vi "SigProc_subVI createPyCode.vi"(0 "newScriptCode":string) -> (1 "scriptStartIdx":i32, 2 "pyCode":string)   [LabVIEW 2018, in "Sig2MS.lvclass"]
uses:
  Sig2MS.lvclass
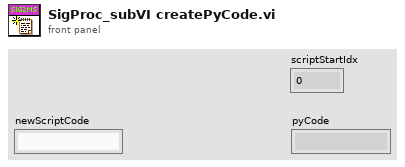
[diagram p1: front panel]
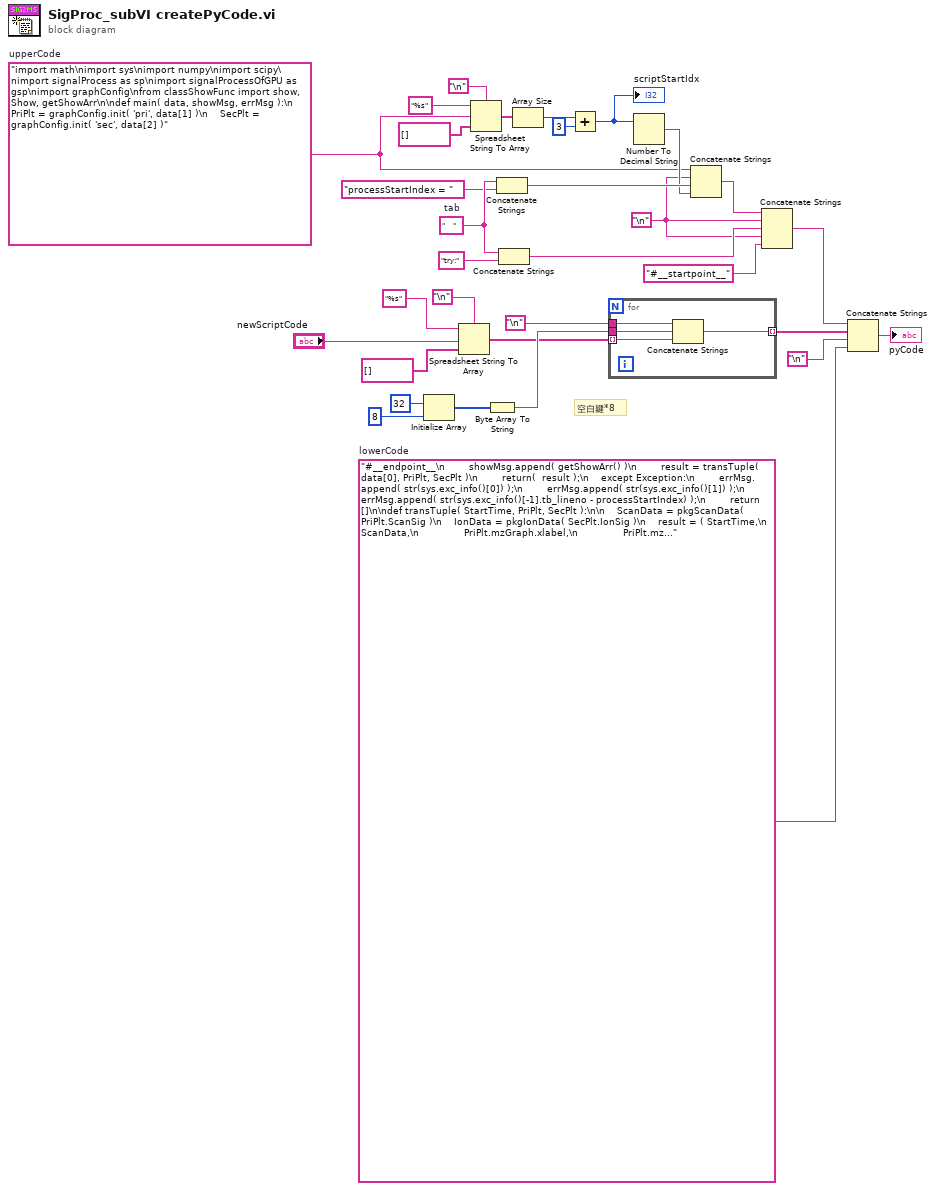
[diagram p0: block diagram]
diagram:
  w14 = "    "  # tab
  w6 = "\n"
  w5 = "#__endpoint__\n        showMsg.append( getShowArr() )\n        result = transTuple( data[0], PriPlt, SecPlt )\n        return(  result );\n    except Exception:\n        errMsg.append( str(sys.exc_info()[0]) );\n        errMsg.append( str(sys.exc_info()[1]) );\n        errMsg.append( str(sys.exc_info()[-1].tb_lineno - processStartIndex) );\n        return []\n\ndef transTuple( StartTime, PriPlt, SecPlt ):\n\n    ScanData = pkgScanData( PriPlt.ScanSig )\n    IonData = pkgIonData( SecPlt.IonSig )\n    result = ( StartTime,\n               ScanData,\n               PriPlt.mzGraph.xlabel,\n               PriPlt.mzGraph.ylabel,\n               PriPlt.tGraph.xlabel,\n               PriPlt.tGraph.ylabel,\n               IonData,\n               SecPlt.ionGraph.xlabel,\n               SecPlt.ionGraph.ylabel )\n    return result\n\ndef pkgScanData( sig ):\n    scanData=[]\n    for sig in sig:\n        if type( sig.xdata ) != list:\n            sig.xdata = sig.xdata.tolist()\n        if type( sig.ydata ) != list:\n            sig.ydata = sig.ydata.tolist()\n            \n        scanTuple = ( sig.dt, sig.xdata, sig.ydata, sig.beta ) \n        scanData.append( scanTuple )\n        \n    return scanData\n\ndef pkgIonData( sig ):\n    ionData=[]\n    for sig in sig:\n        if type( sig.ydata ) != list:\n            sig.ydata = sig.ydata.tolist()\n            \n        ionTuple = ( sig.dt, sig.ydata ) \n        ionData.append( ionTuple )\n\n    return ionData"  # lowerCode
  w3 = "import math\nimport sys\nimport numpy\nimport scipy\nimport signalProcess as sp\nimport signalProcessOfGPU as gsp\nimport graphConfig\nfrom classShowFunc import show, Show, getShowArr\n\ndef main( data, showMsg, errMsg ):\n    PriPlt = graphConfig.init( 'pri', data[1] )\n    SecPlt = graphConfig.init( 'sec', data[2] )"  # upperCode
  # "空白鍵*8"
  n1 = Initialize Array(u8 32, 8 ("dimension size")) -> (w29:u8[])
  n2 = Spreadsheet String To Array(delimiter (Tab)="\n", format string="%s", spreadsheet string="newScriptCode", array type (2D Dbl)=string[] []) -> (array=w24:string[])
  n3 = Spreadsheet String To Array(delimiter (Tab)="\n", format string="%s", spreadsheet string=w3, array type (2D Dbl)=string[] []) -> (array=w16:string[])
  n4 = Byte Array To String(unsigned byte array=w29) -> (string=w28:string)
  n5 = Concatenate Strings(w14, "processStartIndex = " ("string")) -> (w19:string)
  n6 = Concatenate Strings(w14, "try:" ("string")) -> (w20:string)
  n7 = Array Size(array=w16) -> (size(s)=w21:i32)
  n8 = Add(x=w21, y=3) -> (x+y=w1:i32)
  "scriptStartIdx" <- w1
  n9 = for {
    tunnel: w24 -> [w33] mode=indexing
    tunnel: w28 -> [w36]
    tunnel: [w35] -> w23 mode=indexing
    tunnel: "\n" ("delimiter (Tab)") -> [w34]
    n10 = Concatenate Strings(w34, w36, w33) -> (w35:string)
  }
  n11 = Number To Decimal String(number=w1) -> (decimal integer string=w17:string)  [unwired: 1 in]
  n12 = Concatenate Strings(w3, w6, w19, w17) -> (w18:string)
  n13 = Concatenate Strings(w18, w6, w20, w6, "#__startpoint__" ("string")) -> (w8:string)
  n14 = Concatenate Strings(w8, w23, "\n" ("delimiter (Tab)"), w5) -> (→"pyCode":string)
